vi "Z-Scan-Simulation-Analysis.vi"() -> ()   [LabVIEW 2014]
doc: "André Romero - 2016\nandretec@ifsc.usp.br"
uses:
  <vilib>/Utility/file.llb/Write To Spreadsheet File (DBL).vi
  <vilib>/Analysis/NI_AALBase.lvlib
panel:
  out "Dellay VI":u32(graph)=41
  out "Delay DAQ":u32(graph)=205
  in  "number of samples":i32=40000
  in  "rate":dbl=200000.0 format="%#_13g"
  out "variance":dbl format="%0.6f"
  out "standard deviation":dbl format="%0.6f"
  out "mean":dbl format="%0.6f"
  out "Delta voltage":dbl format="%#_8g"
  out "Number of samples":i32=10
  in  "Save ?":bool=TRUE
  in  "delay between points (ms)":u32=100
  out "Z-Scan Graph":dbl[](graph)=[1.112475562979439, 1.1111663496074422, 1.1114924430935662, 1.1133114658150642, 1.1245341570733625, 1.1320445504977776, 1.144878335345933, 1.1549643089236905, 1.179069378705896, 1.232098578163593, 1.3110514938411677, 1.4146614120329504, 1.500625671478743, 1.5859783595669004, 1.6662460956852225, 1.7863376520860226, 1.8169530355197443, 1.8358750604130034, 1.8397621628641059, 1.837506395811384, 1.7951973269741486, 1.5519902542549926, 1.2633724813125091, 1.0477233197591453, 1.0195820625352816, 1.0211275162248006, 1.0214905053215853, 1.0233227228460784, 1.0216737069350172, 1.07200247627774, 1.1975175770487232, 1.353429911922695, 1.453377669857288, 1.5051839925435728, 1.5295770119712113, 1.5298424426553876, 1.5322144570358547, 1.5322243644380145, 1.5328727449574708, 1.533188191269895, 1.5305416563802567, 1.5211116628700019, 1.497615530367908, 1.4554046661930489, 1.4507935840167254, 1.4541395356372617, 1.4516560299793193, 1.4613695583034065, 1.4643873793187043, 1.4627616432837816, 1.4613291676315916, 1.4710692710113442, 1.4583920214175847, 1.4630087118368567, 1.4655746464912016, 1.4622500869081254, 1.465258910145212, 1.470719662657423, 1.460378289599946, 1.4706587197432577, 1.467665843964675, 1.46257555538983, 1.463688392624297, 1.4660121330499556, 1.4652667866600175, 1.458422849363484, 1.4612294585775887, 1.4637617413394435, 1.4681222204425495, 1.4625862387162962, 1.4611468128508411, 1.458952178720894, 1.4682363547454456, 1.4621382423976268, 1.4634620716465216, 1.4613365283410835, 1.4672454190398003, 1.4678275987677105, 1.4641169193061288, 1.4674899822878342, 1.4583075685979272, 1.4635969363653163, 1.4625001041933179, 1.469821670373889, 1.464955952071955, 1.4669013438273408, 1.4649597695257086, 1.460845582627202, 1.4633806646141656, 1.4643919603643532, 1.469557775213437, 1.4625489912968435, 1.4621535785980662, 1.46708956444862, 1.4605931932922538]
  in  "N Points":i32=95
  in  "GO":bool
  out "Z-Scan graph":dbl[][](graph)
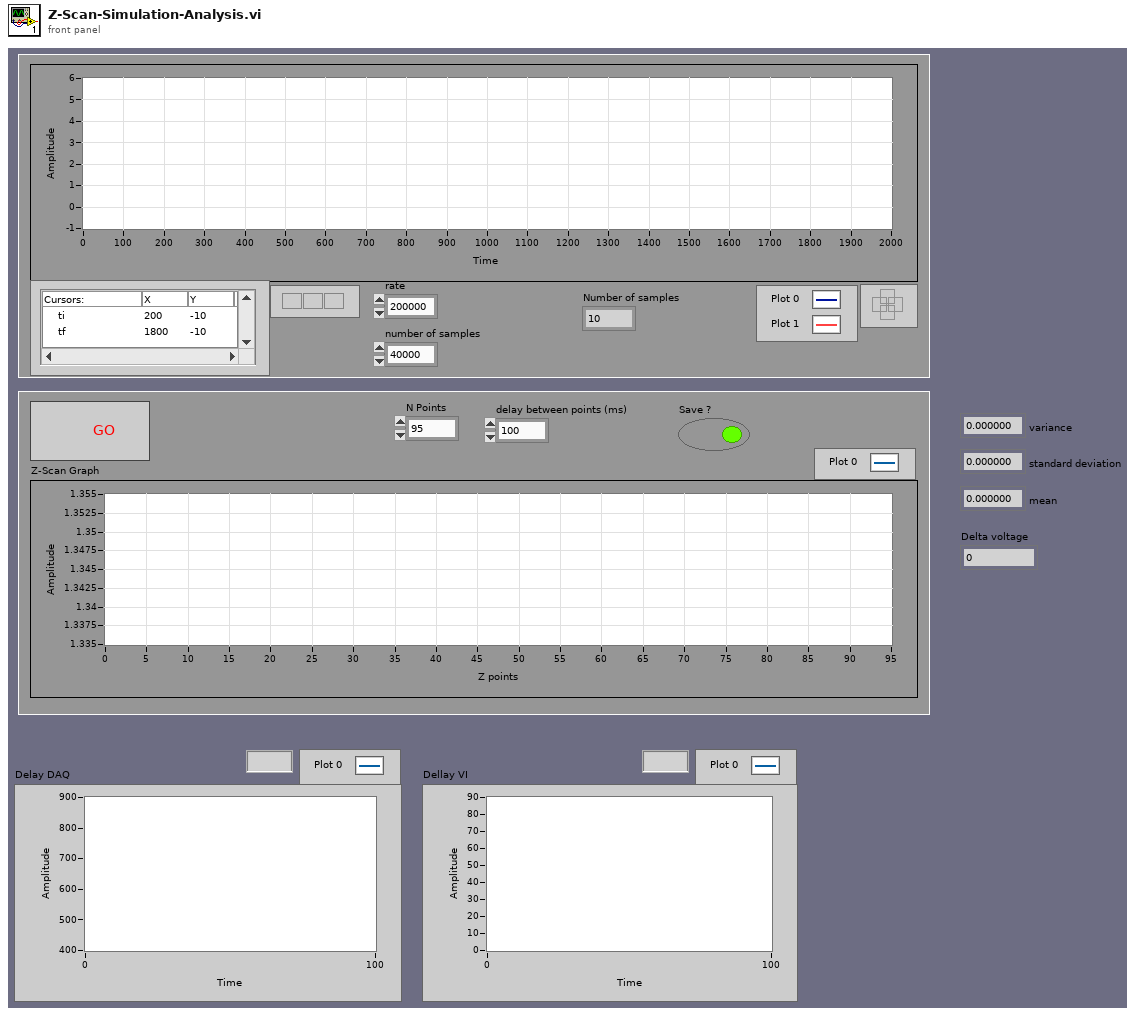
[diagram p1: front panel]
types:
  T1 = typedef "LVCursorListTypeDef.ctl" = cluster{"Name":string, "Color":u32, "Style":u8, "Point Style":u8, "Name Visible":bool, "Allow Drag":bool, "Cursor Mode":u32, "Plot":i32, "Index":i32, "Position":cluster{"X":dbl, "Y":dbl}, "X Scale":u32, "Y Scale":u32, "Watch Plots":i32[], "Watch All Plots":bool, "Plot Area":i32, "Label Offset":cluster{"X":dbl, "Y":dbl}}[]
  T2 = cluster{"Name":string, "Color":u32, "Style":u8, "Point Style":u8, "Name Visible":bool, "Allow Drag":bool, "Cursor Mode":u32, "Plot":i32, "Index":i32, "Position":cluster{"X":dbl, "Y":dbl}, "X Scale":u32, "Y Scale":u32, "Watch Plots":i32[], "Watch All Plots":bool, "Plot Area":i32, "Label Offset":cluster{"X":dbl, "Y":dbl}}
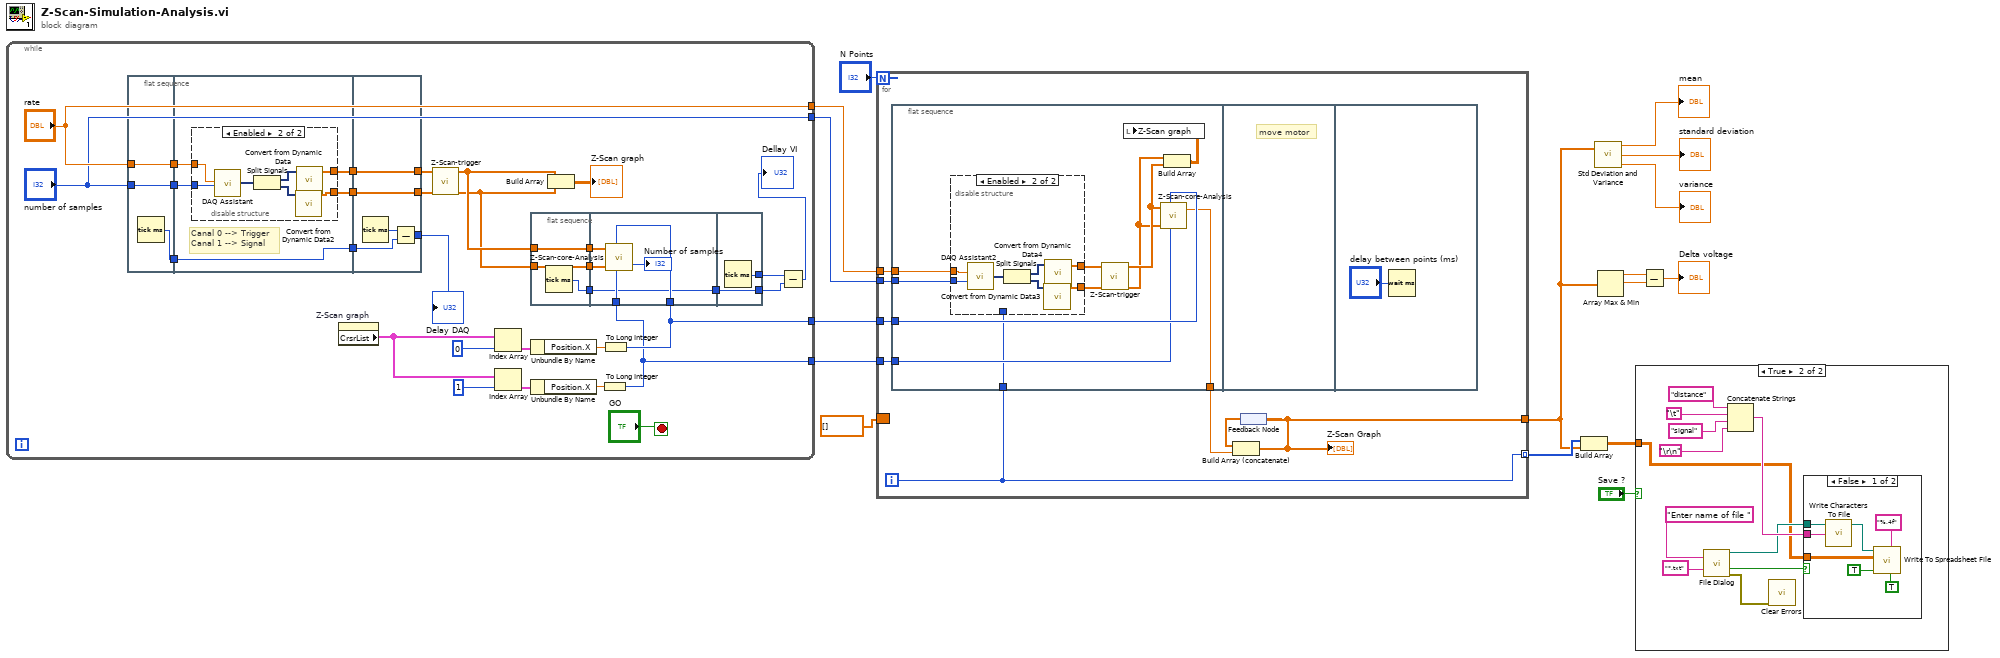
[diagram p0: block diagram]
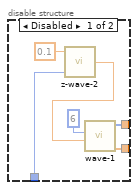
[diagram p2: hidden frame]
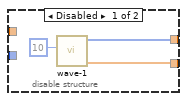
[diagram p3: hidden frame]
diagram:
  n1 = while {
    tunnel: [w38] -> w16
    tunnel: [w37] -> w15
    tunnel: ["rate"] -> w9
    tunnel: ["number of samples"] -> w8
    stop <- "GO" stop-if-true
    n2 = flat-sequence {
      tunnel: "number of samples" -> [w60]
      tunnel: "rate" -> [w61]
      tunnel: [w61] -> w30
      tunnel: [w60] -> w29
      tunnel: [w59] -> w26
      tunnel: w30 -> [w64]
      tunnel: w29 -> [w63]
      tunnel: [w66] -> w28
      tunnel: [w65] -> w27
      tunnel: w26 -> [w62]
      tunnel: [w62] -> w25
      tunnel: [w80] -> w35
      tunnel: [w81] -> w36
      tunnel: w28 -> [w81]
      tunnel: w27 -> [w80]
      tunnel: w25 -> [w78]
      tunnel: [w77] -> w24
      frame #0 {
        n3 = Tick Count (ms)() -> (millisecond timer value=w59:u32)
      }
      frame #1 {
        # "Canal 0 --> Trigger\nCanal 1 --> Signal"
        n4 = disable-structure shown="Enabled" {
          disable-tunnel: [w68 w73] -> w66
          disable-tunnel: [w67 w72] -> w65
          disable-tunnel: w64 -> [_ w76]
          disable-tunnel: w63 -> [_ w75]
          frame Disabled {
            n5 = call "wave-1.vi"("N cycles"=i64 10) -> ("signal"=w67:dbl[], "trigger"=w68:i32[])  [unwired: 7 in]
          }
          frame Enabled {
            n6 = call "DAQ Assistant"("rate"=w76, "number of samples"=w75) -> ("data"=w74:dynamicdata)  [unwired: 15 in, 2 out]
            n7 = Split Signals(w74) -> (w70:dynamicdata, w71:dynamicdata)  [unwired: 2 in]
            n8 = call "Convert from Dynamic Data2"("Dynamic Data Type"=w71) -> ("Array"=w72:dbl[])  [unwired: 3 in]
            n9 = call "Convert from Dynamic Data"("Dynamic Data Type"=w70) -> ("Array"=w73:dbl[])  [unwired: 3 in]
          }
        }
      }
      frame #2 {
        n10 = Tick Count (ms)() -> (millisecond timer value=w79:u32)
        n11 = Subtract(x=w79, y=w78) -> (x-y=w77:u32)
      }
    }
    n12 = property on="Z-Scan graph" class="WFGraph (strict)"() -> ("CrsrList"=w46:T1)  [unwired: 2 in, 2 out]
    n13 = call "Z-Scan-trigger.vi"("signal in"=w35, "trigger in"=w36) -> ("signal out"=w33:dbl[], "trigger out"=w34:dbl[])  [unwired: 5 in, 1 out]
    n14 = Index Array(array=w46, index=0) -> (element=w44:T2)
    n15 = Index Array(array=w46, index=1) -> (element=w43:T2)
    n16 = flat-sequence {
      tunnel: w33 -> [w49]
      tunnel: w34 -> [w50]
      tunnel: [w50] -> w23
      tunnel: [w49] -> w22
      tunnel: [w48] -> w20
      tunnel: w38 -> [w55]
      tunnel: w37 -> [w54]
      tunnel: w23 -> [w53]
      tunnel: w22 -> [w52]
      tunnel: w20 -> [w51]
      tunnel: [w51] -> w19
      tunnel: [w58] -> w21
      tunnel: w19 -> [w57]
      tunnel: [w57] -> w18
      frame #0 {
        n17 = Tick Count (ms)() -> (millisecond timer value=w48:u32)
      }
      frame #1 {
        n18 = call "Z-Scan-core-Analysis.vi"("trigger in"=w53, "ti"=w55, "signal in"=w52, "tf"=w54) -> ("number of samples"=→"Number of samples":i32)  [unwired: 1 in, 1 out]
      }
      frame #2 {
        n19 = Tick Count (ms)() -> (millisecond timer value=w58:u32)
      }
    }
    n20 = Unbundle By Name(w44) -> ("Position.X"=w42:dbl)
    n21 = Unbundle By Name(w43) -> ("Position.X"=w41:dbl)
    n22 = Build Array(w33, w34) -> (→"Z-Scan graph":dbl[][])
    n23 = To Long Integer(number=w41) -> (32bit integer=w37:i32)
    n24 = To Long Integer(number=w42) -> (32bit integer=w38:i32)
    n25 = Subtract(x=w21, y=w18) -> (x-y=→"Dellay VI":u32)
    "Delay DAQ" <- w24
  }
  n26 = for {
    N: "N Points" -> [_]
    tunnel: w16 -> [w89]
    tunnel: w15 -> [w88]
    tunnel: [w85] -> w14 mode=indexing
    border: dbl[] [] -> [_]
    tunnel: [w84] -> w1
    tunnel: w9 -> [w83]
    tunnel: w8 -> [w82]
    i -> [w85]
    n27 = flat-sequence {
      tunnel: w89 -> [w100]
      tunnel: w88 -> [w99]
      tunnel: [w98] -> w86
      tunnel: w85 -> [w92]
      tunnel: w83 -> [w91]
      tunnel: w82 -> [w90]
      frame #0 {
        n28 = disable-structure shown="Enabled" {
          disable-tunnel: [w106 w110] -> w97
          disable-tunnel: [w105 w109] -> w96
          disable-tunnel: w92 -> [w101 _]
          disable-tunnel: w91 -> [_ w108]
          disable-tunnel: w90 -> [_ w107]
          frame Disabled {
            n29 = call "z-wave-2.vi"("index"=w101, "amplitutude"=0.1) -> ("element"=w102:dbl)  [unwired: 1 in, 2 out]
            n30 = call "wave-1.vi"("slope"=w102, "N cycles"=i64 6) -> ("signal"=w105:dbl[], "trigger"=w106:i32[])  [unwired: 6 in]
          }
          frame Enabled {
            n31 = call "DAQ Assistant2"("rate"=w108, "number of samples"=w107) -> ("data"=w111:dynamicdata)  [unwired: 15 in, 2 out]
            n32 = Split Signals(w111) -> (w113:dynamicdata, w112:dynamicdata)  [unwired: 2 in]
            n33 = call "Convert from Dynamic Data3"("Dynamic Data Type"=w112) -> ("Array"=w109:dbl[])  [unwired: 3 in]
            n34 = call "Convert from Dynamic Data4"("Dynamic Data Type"=w113) -> ("Array"=w110:dbl[])  [unwired: 3 in]
          }
        }
        n35 = call "Z-Scan-trigger.vi"("signal in"=w96, "trigger in"=w97) -> ("signal out"=w93:dbl[], "trigger out"=w94:dbl[])  [unwired: 5 in, 1 out]
        n36 = call "Z-Scan-core-Analysis.vi"("trigger in"=w94, "ti"=w100, "signal in"=w93, "tf"=w99) -> ("mean tf/ti"=w98:dbl)  [unwired: 1 in, 1 out]
        n37 = Build Array(w93, w94) -> (w95:dbl[][])
        n38 = local write "Z-Scan graph"(w95) -> ()
      }
      frame #1 {
        # "move motor"
      }
      frame #2 {
        n39 = Wait (ms)(milliseconds to wait="delay between points (ms)") -> ()  [unwired: 1 out]
      }
    }
    n40 = feedback #1() -> (w87:dbl[])
    n41 = Build Array (concatenate)(w87, w86) -> (w84:dbl[])
    "Z-Scan Graph" <- w84
    n42 = feedback-in #1(w84) -> ()
  }
  n43 = Build Array(w14, w1) -> (w12:dbl[][])
  n44 = call <vilib>:"Std Deviation and Variance.vi"("X"=w1) -> ("mean"=→"mean":dbl, "standard deviation"=→"standard deviation":dbl, "variance"=→"variance":dbl)  [unwired: 1 in]
  n45 = Array Max & Min(array=w1) -> (max value=w7:dbl, min value=w6:dbl)  [unwired: 2 out]
  n46 = case shown="True" "Save ?" {
    tunnel: w12 -> [_ w118]
    frame False {
    }
    frame True {
      n47 = call "File Dialog"("prompt"="Enter name of file ", "pattern (all files)"="*.txt") -> ("selected path"=w121:path, "cancelled"=w123:bool, "error out"=w122:errorcluster)  [unwired: 10 in, 1 out]
      n48 = Concatenate Strings("distance", "\t", "signal", "\r\n") -> (w125:string)
      n49 = call <vilib>:"Clear Errors.vi"("error in (no error)"=w122) -> ()  [unwired: 5 in, 2 out]
      n50 = case shown="False" w123 {
        tunnel: w121 -> [w132 _]
        tunnel: w118 -> [w129 _]
        tunnel: w125 -> [w128 _]
        frame False {
          n51 = call <vilib>:"Write Characters To File.vi"("character string"=w128, "file path (dialog if empty)"=w132) -> ("new file path (Not A Path if cancelled)"=w131:path)  [unwired: 3 in]
          n52 = call-poly <vilib>:"Write To Spreadsheet File.vi"("transpose? (no:F)"=TRUE, "format (%.3f)"="%.4f", "append to file? (new file:F)"=TRUE, "2D data"=w129, "file path (dialog if empty)"=w131) -> ()  [unwired: 3 in, 1 out]
        }
        frame True {
        }
      }
    }
  }
  n53 = Subtract(x=w7, y=w6) -> (x-y=→"Delta voltage":dbl)
